vi "MCSGlobalVars.vi"() -> ()   [LabVIEW 2014]
uses:
  Controls/MCSstate.ctl
panel:
  in  "errorCount":i8
  in  "MCSstate":T1
  in  "nOfBunches":i32
  in  "nOfBins":u32
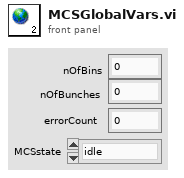
[diagram p1: front panel]
types:
  T1 = typedef "MCSstate.ctl" = enum16{"idle", "scanning", "done", "error"}
diagram:
